vi "Bus Arming Cancel.vi"(8 "error in (no error)":errorcluster, 11 "VISA resource name":refnum<visa-resource-name>) -> (0 "error out":errorcluster, 3 "VISA resource name out":refnum<visa-resource-name>)   [LabVIEW 2019, in "Pendulum CNT90.lvlib"]
doc: "Overrides the waiting for bus arm, provided the source is set to bus. When this command is issued, the counter will immediately exit the “wait-for-busarm” state. The counter generates an error if it receives this command when the trigger subsystem is not in the “wait-for-bus-arm” state. If the Arming source is set to Immediate, this command is ignored."
uses:
  Pendulum CNT90.lvlib
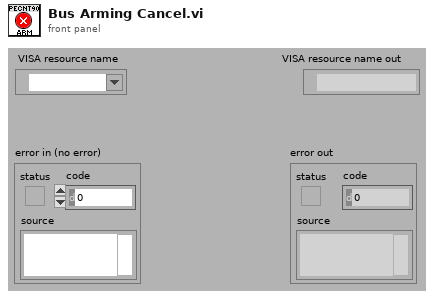
[diagram p1: front panel]
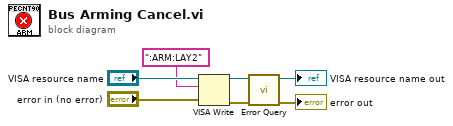
[diagram p0: block diagram]
diagram:
  n1 = VISA Write(VISA resource name="VISA resource name", write buffer=":ARM:LAY2", error in (no error)="error in (no error)") -> (VISA resource name out=w5:refnum<visa-resource-name>, error out=w2:errorcluster)  [unwired: 1 out]
  n2 = call "Error Query.vi"("error in (no error)"=w2, "VISA resource name"=w5) -> ("error out"=→"error out":errorcluster, "VISA resource name out"=→"VISA resource name out":refnum<visa-resource-name>)  [unwired: 6 in, 2 out]
